vi "processData.vi"(8 "error in (no error)":errorcluster, 10 "model":refnum<class "Model.lvclass">, 11 "RampingUpPressurePState in":refnum<class "RampingUpPressurePState.lvclass">) -> (0 "error out":errorcluster, 2 "model 2":refnum<class "Model.lvclass">, 3 "RampingUpPressurePState out":refnum<class "RampingUpPressurePState.lvclass">)   [LabVIEW 2015, in "RampingUpPressurePState.lvclass"]
uses:
  RampingUpPressurePState.lvclass
  Model/Model/Model.lvclass
  PreconditioningState/PreconditioningState.lvclass
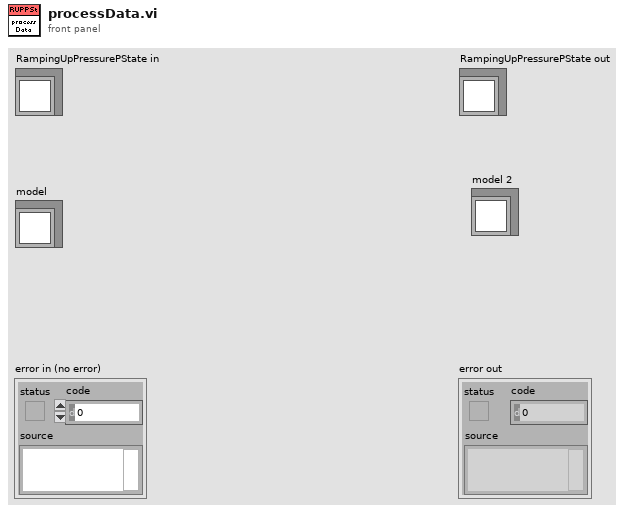
[diagram p1: front panel]
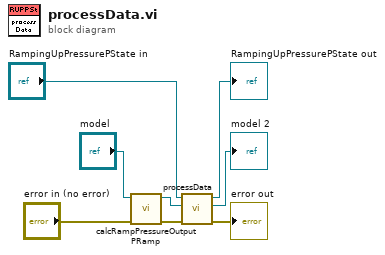
[diagram p0: block diagram]
diagram:
  n1 = call "calcRampPressureOutputPRamp.vi"("error in (no error)"="error in (no error)", "Model in"="model") -> ("error out"=w1:errorcluster, "Model out"=w3:refnum<class "Model.lvclass">)  [unwired: 8 in]
  n2 = call-parent "processData.vi"("error in (no error)"=w1, "model"=w3, "TestingState in"="RampingUpPressurePState in") -> ("error out"=→"error out":errorcluster, "model 2"=→"model 2":refnum<class "Model.lvclass">, "TestingState out"=→"RampingUpPressurePState out":refnum<class "RampingUpPressurePState.lvclass">)  [unwired: 6 in]
